vi "PXI-Create DIO Tasks.vi"(0 "Sync Task":T1, 11 "error in (no error)":errorcluster) -> (2 "DI Tasks":T1[](array[typedef]), 3 "DO Tasks":T1[](array[typedef]), 15 "error out":errorcluster)   [LabVIEW 2020]
uses:
  Type Defs/Task Struct.ctl
  PXI Globals.vi
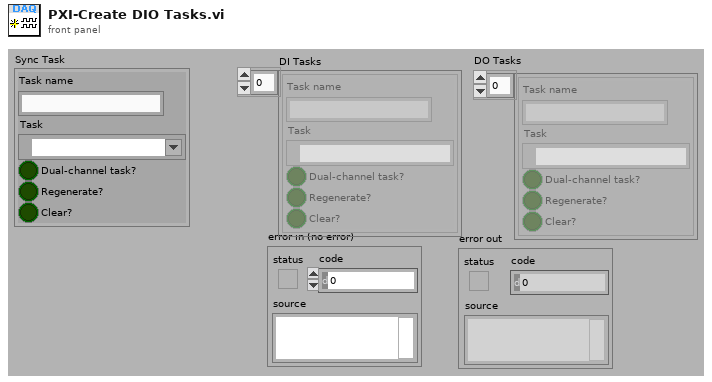
[diagram p1: front panel]
types:
  T1 = typedef "Task Struct.ctl" = cluster{"Task name":string, "Task":refnum<k21>, "Dual-channel task?":bool, "Regenerate?":bool, "Clear?":bool}
  T2 = typedef "DI Channel Struct.ctl" = cluster{"Physical Channel":tag, "Channel Num":i32[]}
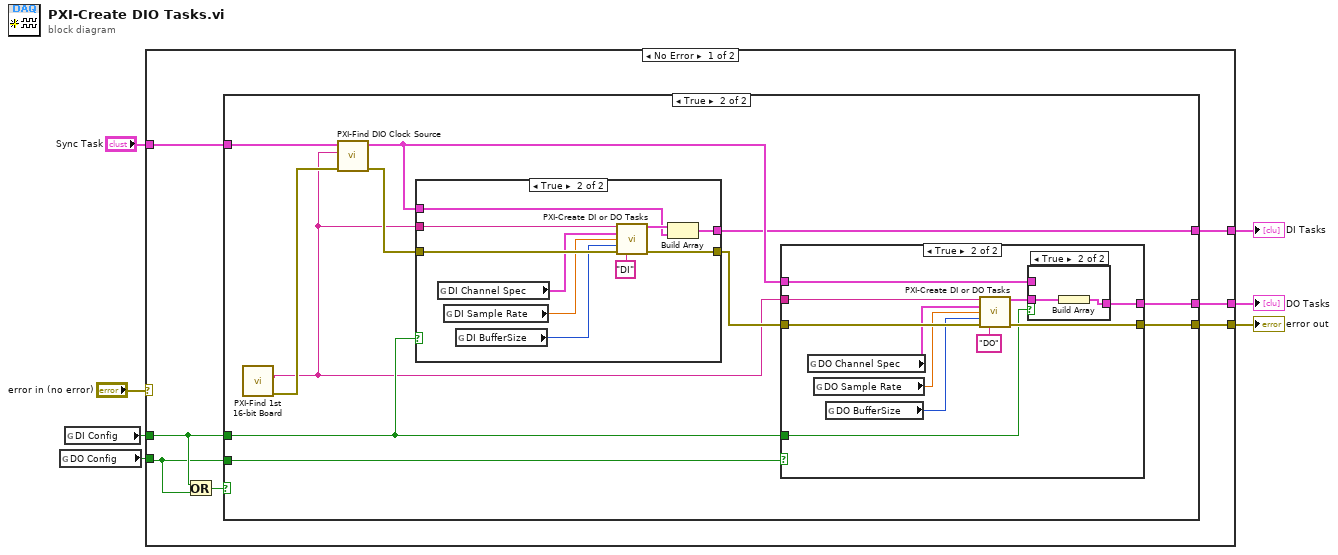
[diagram p0: block diagram]
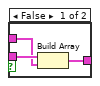
[diagram p4: hidden frame]
diagram:
  n1 = global read "PXI Globals.vi" "DO Config"() -> (w2:bool)
  n2 = global read "PXI Globals.vi" "DI Config"() -> (w5:bool)
  n3 = case shown="No Error" "error in (no error)" {
    selector: "error in (no error)" -> [_ w54]
    tunnel: [w14 _] -> w4
    tunnel: [w13 w54] -> w7
    tunnel: w5 -> [w10 _]
    tunnel: "Sync Task" -> [w12 _]
    tunnel: w2 -> [w9 _]
    tunnel: [w8 _] -> w1
    frame No Error {
      n4 = Or(x=w10, y=w9) -> (x .or. y?=w11:bool)
      n5 = case shown="True" w11 {
        tunnel: [_ w21] -> w14
        tunnel: [_ w18] -> w13
        tunnel: w12 -> [_ w25]
        tunnel: w10 -> [_ w19]
        tunnel: w9 -> [_ w20]
        tunnel: [_ w17] -> w8
        frame False {
        }
        frame True {
          n6 = call "PXI-Find 1st 16-bit Board.vi"() -> ("error out"=w16:errorcluster, "DAQmx Device Name"=w15:tag)  [unwired: 9 in, 1 out]
          n7 = call "PXI-Find DIO Clock Source.vi"("error in (no error)"=w16, "DAQmx Device Name"=w15, "Sync Task"=w25) -> ("error out"=w24:errorcluster, "Counter Task"=w23:T1)  [unwired: 7 in]
          n8 = case shown="True" w19 {
            tunnel: w24 -> [w43 w53]
            tunnel: w15 -> [_ w52]
            tunnel: [w43 w48] -> w22
            tunnel: [_ w46] -> w21
            tunnel: w23 -> [_ w45]
            frame False {
            }
            frame True {
              n9 = global read "PXI Globals.vi" "DI Channel Spec"() -> (w51:T2)
              n10 = global read "PXI Globals.vi" "DI Sample Rate"() -> (w50:dbl)
              n11 = global read "PXI Globals.vi" "DI BufferSize"() -> (w49:i32)
              n12 = call "PXI-Create DI or DO Tasks.vi"("DAQmx Device Name"=w52, "Channel Spec"=w51, "Sample Rate"=w50, "Buffer Size"=w49, "error in"=w53, "Task name"="DI") -> ("Task"=w47:T1, "error out"=w48:errorcluster)  [unwired: 8 in]
              n13 = Build Array(w47, w45) -> (w46:T1[])
            }
          }
          n14 = case shown="True" w20 {
            tunnel: w22 -> [w26 w37]
            tunnel: w15 -> [_ w36]
            tunnel: [w26 w32] -> w18
            tunnel: [_ w30] -> w17
            tunnel: w23 -> [_ w29]
            tunnel: w19 -> [_ w28]
            frame False {
            }
            frame True {
              n15 = global read "PXI Globals.vi" "DO Channel Spec"() -> (w35:T2)
              n16 = global read "PXI Globals.vi" "DO Sample Rate"() -> (w34:dbl)
              n17 = global read "PXI Globals.vi" "DO BufferSize"() -> (w33:i32)
              n18 = call "PXI-Create DI or DO Tasks.vi"("DAQmx Device Name"=w36, "Channel Spec"=w35, "Sample Rate"=w34, "Buffer Size"=w33, "error in"=w37, "Task name"="DO") -> ("Task"=w31:T1, "error out"=w32:errorcluster)  [unwired: 8 in]
              n19 = case shown="True" w28 {
                tunnel: w31 -> [w40 w42]
                tunnel: [w39 w41] -> w30
                tunnel: w29 -> [w38 _]
                frame False {
                  n20 = Build Array(w40, w38) -> (w39:T1[])
                }
                frame True {
                  n21 = Build Array(w42) -> (w41:T1[])
                }
              }
            }
          }
        }
      }
    }
    frame Error {
    }
  }
  "error out" <- w7
  "DI Tasks" <- w4
  "DO Tasks" <- w1
